vi "create-time-array.vi"(0 "Invert":bool=TRUE, 2 "Array Size":i32, 3 "dt":dbl, 4 "t0":dbl) -> (1 "Time Array":dbl[](array[numeric]))   [LabVIEW 2017]
panel:
  out "Array Plot":cluster{"Y":dbl[], "Y":dbl[]}[](graph)
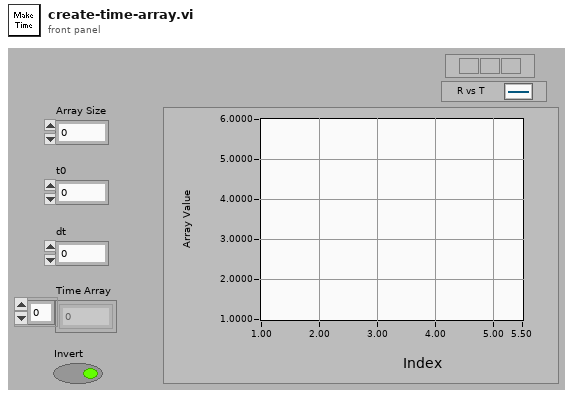
[diagram p1: front panel]
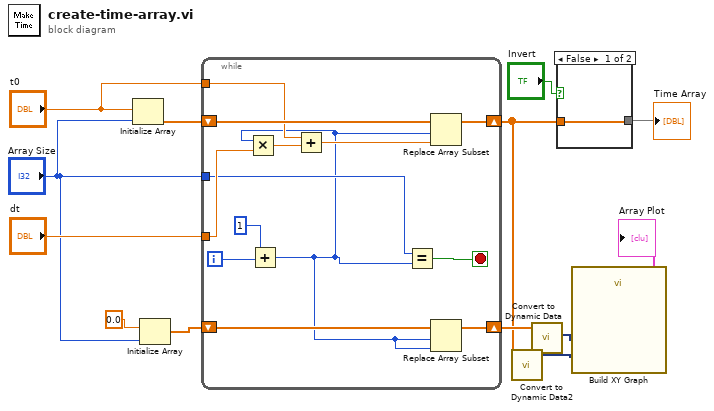
[diagram p0: block diagram]
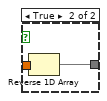
[diagram p2: hidden frame]
diagram:
  n1 = Initialize Array("t0", "Array Size") -> (w13:dbl[])
  n2 = Initialize Array(0.0, "Array Size") -> (w6:dbl[])
  n3 = while {
    tunnel: "dt" -> [w25]
    shift-right: [w22] -> w3
    shift-left: w13 -> [w26]
    tunnel: "Array Size" -> [w24]
    tunnel: "t0" -> [w18]
    shift-right: [w15] -> w5
    shift-left: w6 -> [w16]
    i -> [w20]
    stop <- w23 stop-if-true
    n4 = Add(x=1, y=w20) -> (x+y=w14:i32)
    n5 = Multiply(x=w14, y=w25) -> (x*y=w19:dbl)
    n6 = Add(x=w18, y=w19) -> (x+y=w17:dbl)
    n7 = Equal?(x=w24, y=w14) -> (x = y?=w23:bool)
    n8 = Replace Array Subset(array=w26, new element=w17, index=w14) -> (w22:dbl[])
    n9 = Replace Array Subset(array=w16, new element=w14, index=w14) -> (w15:dbl[])
  }
  n10 = call "Convert to Dynamic Data2"("Array"=w3) -> ("Dynamic Data Type"=w11:dynamicdata)  [unwired: 3 in]
  n11 = call "Convert to Dynamic Data"("Array"=w5) -> ("Dynamic Data Type"=w4:dynamicdata)  [unwired: 3 in]
  n12 = case shown="False" "Invert" {
    tunnel: w3 -> [w27 w29]
    tunnel: [w27 w28] -> w2
    frame False {
    }
    frame True {
      n13 = Reverse 1D Array(array=w29) -> (reversed array=w28:dbl[])
    }
  }
  "Time Array" <- w2
  n14 = call "Build XY Graph"("Y Input"=w11, "X Input"=w4) -> ("XY Graph"=→"Array Plot":cluster{"Y":dbl[], "Y":dbl[]}[])  [unwired: 3 in, 6 out]
